vi "picoquant_receive_buffer.vi"(8 "error in (no error)":errorcluster, 11 "picoquant_generic in":refnum<class "picoquant_generic.lvclass">) -> (0 "error out":errorcluster, 1 "queue_timed_out":bool, 2 "data":u32[](array[numeric]), 3 "picoquant_generic out":refnum<class "picoquant_generic.lvclass">)   [LabVIEW 2015, in "picoquant_generic.lvclass"]
uses:
  picoquant_generic.lvclass
  picoquant_generic.lvclass/picoquant_generic.ctl
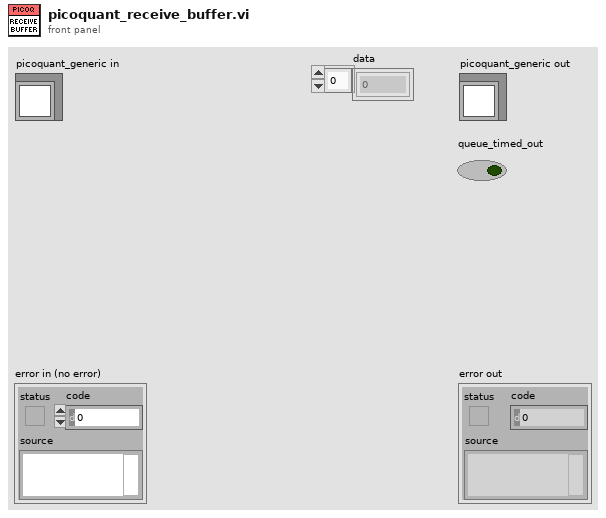
[diagram p1: front panel]
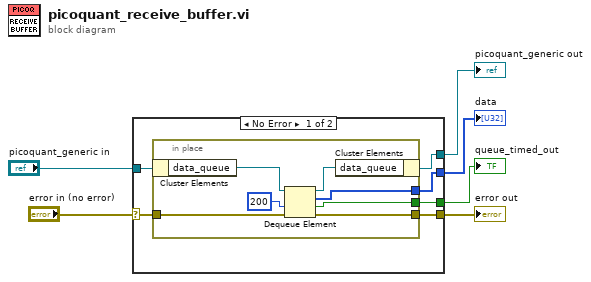
[diagram p0: block diagram]
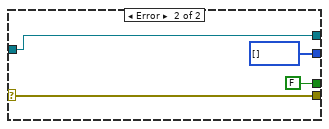
[diagram p2: hidden frame]
diagram:
  n1 = case shown="No Error" "error in (no error)" {
    selector: "error in (no error)" -> [w11 w23]
    tunnel: [w8 w23] -> w5
    tunnel: [w7 w22] -> w3
    tunnel: "picoquant_generic in" -> [w12 w22]
    tunnel: [w10 FALSE ("timed out?")] -> w2
    tunnel: [w9 u32[] [] ("data")] -> w1
    frame No Error {
      n2 = in-place {
        in-place-border: w11 -> [w17]
        in-place-border: [w15] -> w10
        in-place-border: [w14] -> w9
        in-place-border: [w13] -> w8
        n3 = in-place-cluster #1(w12) -> ("data_queue"=w19:refnum<queue>)
        n4 = Dequeue Element(queue=w19, timeout in ms (-1)=200, error in (no error)=w17) -> (queue out=w16:refnum<queue>, element=w14:u32[], timed out?=w15:bool, error out=w13:errorcluster)
        n5 = in-place-cluster #1("data_queue"=w16) -> (w7:refnum<class "picoquant_generic.lvclass">)
      }
    }
    frame Error {
    }
  }
  "error out" <- w5
  "picoquant_generic out" <- w3
  "queue_timed_out" <- w2
  "data" <- w1
